vi "Write Dependencies.vi"(8 "error in (no error)":errorcluster, 9 "Control Experiment":refnum<class "Control Experiment.lvclass">, 10 "SweepControl":refnum<class "SweepControl.lvclass">, 11 "Transport in":refnum<class "Transport.lvclass">) -> (0 "error out":errorcluster, 3 "Transport out":refnum<class "Transport.lvclass">)   [LabVIEW 2016, in "Transport.lvclass"]
uses:
  Transport.lvclass
  SweepControl/SweepControl.lvclass
  Control Experiment/Control Experiment.lvclass
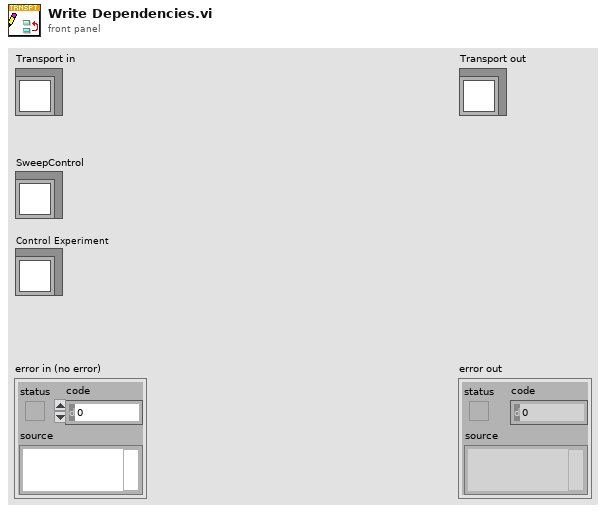
[diagram p1: front panel]
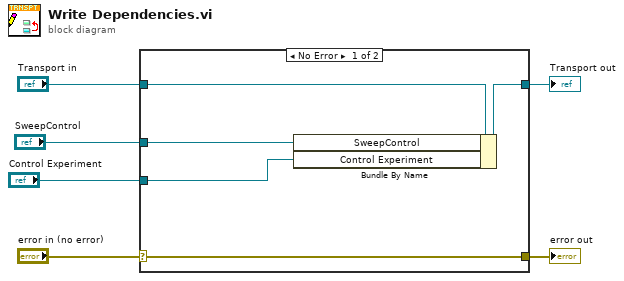
[diagram p0: block diagram]
diagram:
  n1 = case shown="No Error" "error in (no error)" {
    selector: "error in (no error)" -> [w7 w12]
    tunnel: [w7 w12] -> w5
    tunnel: [w10 w13] -> w3
    tunnel: "Transport in" -> [w11 w13]
    tunnel: "SweepControl" -> [w9 _]
    tunnel: "Control Experiment" -> [w8 _]
    frame No Error {
      n2 = Bundle By Name(cluster=w11, "SweepControl"=w9, "Control Experiment"=w8) -> (w10:refnum<class "Transport.lvclass">)
    }
    frame Error {
    }
  }
  "error out" <- w5
  "Transport out" <- w3
